vi "TSM SSC Digital Burst Pattern [Pass Fail].vi"(0 "Digital TSM In":T1, 1 "Start Label":string, 2 "select digital function?":bool=TRUE caption="select digital function? (T)", 7 "timeout (s)":dbl=10.0, 11 "error in":errorcluster) -> (4 "Digital TSM out":T1, 6 "Per-Site Pass":bool[](array[boolean]), 15 "error out":errorcluster)   [LabVIEW 2019]
doc: "Uses the start label you specify to burst the pattern on the pin(s) and pin group(s) you specify, waits for the burst to complete, and returns per-site pass/fail results."
uses:
  TSM/TSM SSC Digital.ctl
  <vilib>/NI_TestStand_SemiconductorModule/NI_TestStand_Semiconductor_Module.lvlibp/PinMap/Digital Pattern/PinQueryContext/DigitalPatternPinQueryContext.lvclass
  SSC Digital/SSC Digital.ctl
  b5bdf898-0a80-4460-9acf-d5bdb82107c7.vi
  Shared SubVIs/Site List to Site Numbers.vi
  Shared SubVIs/Trim Whitespace [Inlined].vi
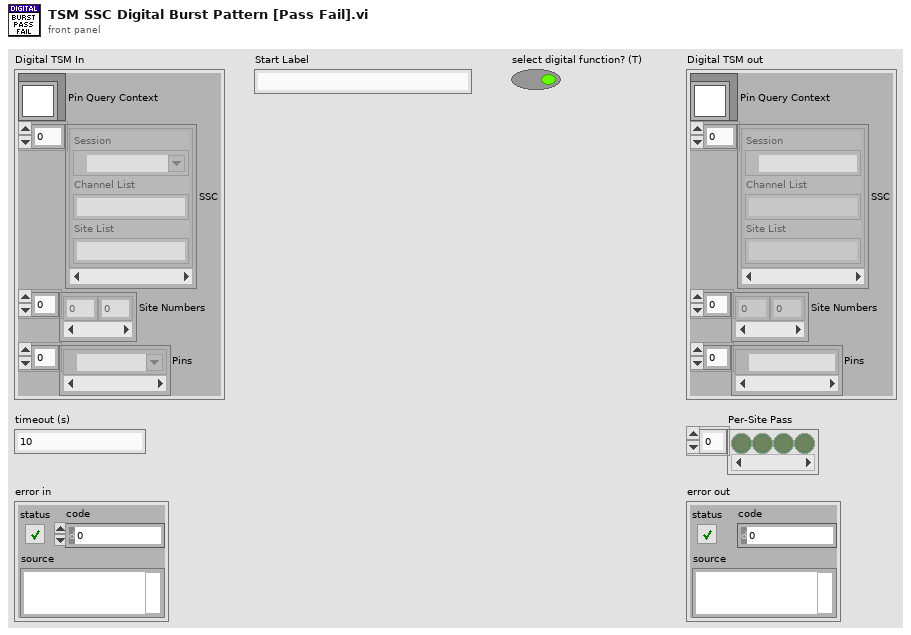
[diagram p1: front panel]
types:
  T1 = typedef "TSM SSC Digital.ctl" = cluster{"Pin Query Context":refnum<class "DigitalPatternPinQueryContext.lvclass">, "SSC":T2[], "Site Numbers":i32[], "Pins":tag[]}
  T2 = typedef "SSC Digital.ctl" = cluster{"Session":refnum<k15>, "Channel List":string, "Site List":string}
  T3 = typedef "Digital 1D Location Array in a Cluster.ctl" = cluster{"Digital 1D Location Array":i32[]}
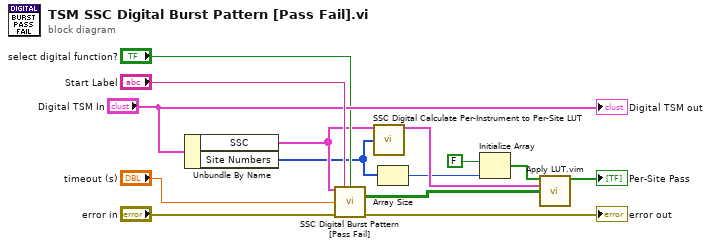
[diagram p0: block diagram]
diagram:
  n1 = Unbundle By Name("Digital TSM In") -> ("SSC"=w9:T2[], "Site Numbers"=w5:i32[])
  n2 = call "SSC Digital Burst Pattern [Pass Fail].vi"("Digital SSC in"=w9, "Start Label"="Start Label", "select digital function?"="select digital function?", "timeout (s)"="timeout (s)", "error in"="error in") -> ("Per-Instrument Pass"=w8:bool[][], "error out"=→"error out":errorcluster)  [unwired: 8 in, 1 out]
  n3 = call "SSC Digital Calculate Per-Instrument to Per-Site LUT.vi"("Digital SSC In"=w9, "Sites"=w5) -> ("Per-Instrument to Per-Site LUT"=w7:T3[])  [unwired: 13 in]
  n4 = Array Size(array=w5) -> (size(s)=w4:i32)
  n5 = Initialize Array(FALSE, w4) -> (w2:bool[])
  n6 = call "Apply LUT.vim"("Initialized Array"=w2, "LUT"=w7, "Results to Apply LUT to"=w8) -> ("Array Out"=→"Per-Site Pass":bool[])  [unwired: 12 in]
  "Digital TSM out" <- "Digital TSM In"
